vi "getObjectPrivateData.vi"(8 "error in (no error)":errorcluster, 10 "object in":refnum<class>) -> (0 "error out":errorcluster, 3 "privateData":variant[](array[variant]), 5 "classNames":string[](array[string]))   [LabVIEW 2020, in "openg_variant.lvlib" / "Reflection.lvclass"]
doc: "This VI returns the class names, and private data values for the class hierarchy (top to bottom) of the input object. \n\nGCraftsman JSON Object Serialization Toolkit\nwww.GCraftsman.com\nCopyright (c) 2017, GCraftsman"
uses:
  Reflection.lvclass
panel:
  # "EXPERIMENTAL"
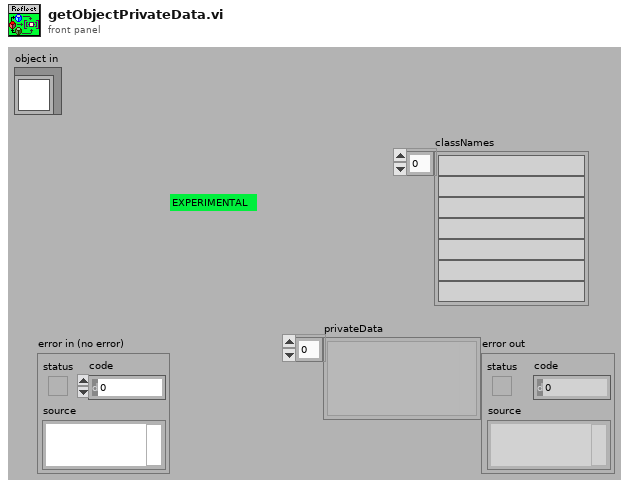
[diagram p1: front panel]
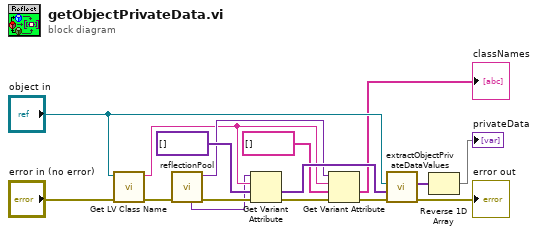
[diagram p0: block diagram]
diagram:
  n1 = call <vilib>:"Get LV Class Name.vi"("error in (no error)"="error in (no error)", "object"="object in") -> ("error out"=w4:errorcluster, "class name"=w10:string)  [unwired: 8 in]
  n2 = call "reflectionPool.vi"("error in (no error)"=w4) -> ("error out"=w5:errorcluster, "classHierarchyLUT"=w11:variant, "classPrivateDataLUT"=w1:variant)  [unwired: 5 in, 3 out]
  n3 = Get Variant Attribute(Variant=w1, name=w10, default value (empty Variant)=variant[] [], error in=w5) -> (value=w12:variant[], error out=w6:errorcluster)  [unwired: 2 out]
  n4 = Get Variant Attribute(Variant=w11, name=w10, default value (empty Variant)=string[] [] ("classNames"), error in=w6) -> (value=→"classNames":string[], error out=w7:errorcluster)  [unwired: 2 out]
  n5 = call "extractObjectPrivateDataValues.vi"("error in (no error)"=w7, "classPrivateDataDefaults"=w12, "Object in"="object in") -> ("error out"=→"error out":errorcluster, "objectPrivateData"=w16:variant[])  [unwired: 6 in]
  n6 = Reverse 1D Array(array=w16) -> (reversed array=→"privateData":variant[])
